vi "lqSetManifestation.vi"(8 "Error In":errorcluster, 10 "Manifestation":string, 11 "LQSerialData in":refnum<class "LQSerialData.lvclass">) -> (0 "Error Out":errorcluster, 3 "LQSerialData out":refnum<class "LQSerialData.lvclass">)   [LabVIEW 2013, in "Template.lvlib" / "LQSerialData.lvclass"]
uses:
  LQSerialData.lvclass
  LQSerialData.lvclass/LQSerialData.ctl
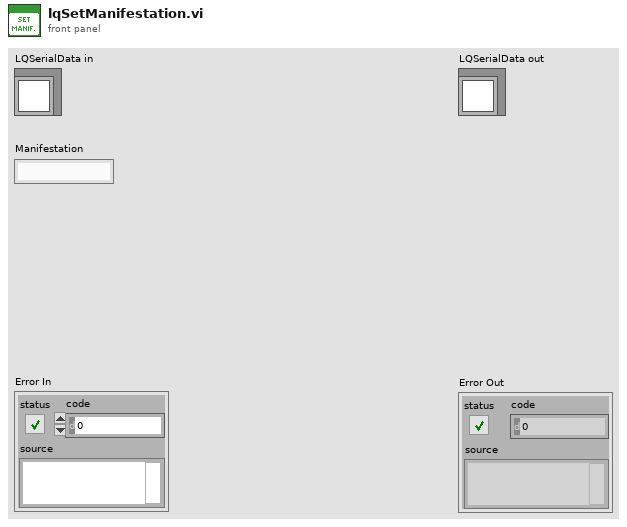
[diagram p1: front panel]
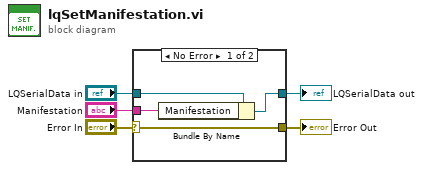
[diagram p0: block diagram]
diagram:
  n1 = case shown="No Error" "Error In" {
    selector: "Error In" -> [w6 w10]
    tunnel: "LQSerialData in" -> [w9 w11]
    tunnel: [w8 w11] -> w4
    tunnel: "Manifestation" -> [w7 _]
    tunnel: [w6 w10] -> w1
    frame No Error {
      n2 = Bundle By Name(cluster=w9, "Manifestation"=w7) -> (w8:refnum<class "LQSerialData.lvclass">)
    }
    frame Error {
    }
  }
  "LQSerialData out" <- w4
  "Error Out" <- w1
